vi "Call Matlab Function.vi"(7 "Timestamp":bool, 8 "error in (no error)":errorcluster, 9 "Matlab Param Array":cluster{"Name":string, "Data":variant}[](array[cluster]), 10 "Function name":string="netStartTrial", 11 "TrialBasedExperiment in":refnum<class "MatlabExperiment.lvclass">) -> (0 "error out":errorcluster, 1 "Return value struct":cluster{"Name":string, "Data":variant}[](array[cluster]), 2 "Return value I32":i32, 3 "TrialBasedExperiment out":refnum<class "MatlabExperiment.lvclass">)   [LabVIEW 2010, in "MatlabExperiment.lvclass"]
uses:
  MatlabExperiment.lvclass
  Matlab API/Matlab API.lvlib
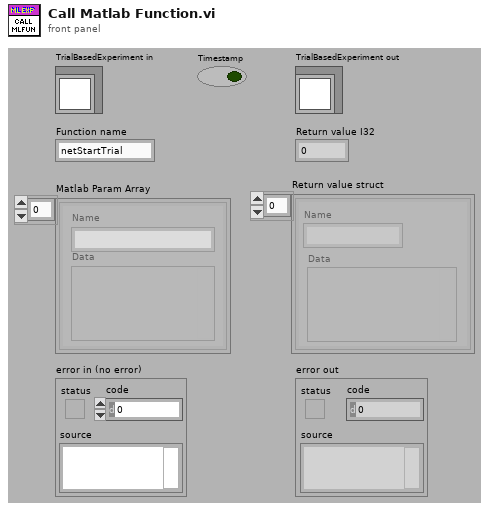
[diagram p1: front panel]
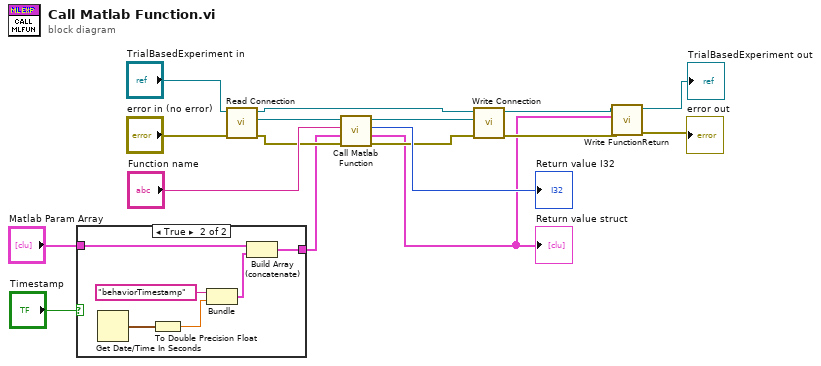
[diagram p0: block diagram]
diagram:
  n1 = case shown="True" "Timestamp" {
    tunnel: "Matlab Param Array" -> [w18 w22]
    tunnel: [w18 w21] -> w7
    frame False {
    }
    frame True {
      n2 = Get Date/Time In Seconds() -> (seconds since 1Jan1904=w20:timestamp)
      n3 = To Double Precision Float(number=w20) -> (double precision float=w19:dbl)
      n4 = Bundle("behaviorTimestamp", w19) -> (w23:cluster{string, dbl})  [unwired: 1 out]
      n5 = Build Array (concatenate)(w22, w23) -> (w21:cluster{"Name":string, "Data":variant}[])
    }
  }
  n6 = call-dynamic "Read Connection.vi"("error in (no error)"="error in (no error)", "TrialBasedExperiment in"="TrialBasedExperiment in") -> ("error out"=w13:errorcluster, "Connection"=w15:refnum<k5>, "TrialBasedExperiment out"=w17:refnum<class "MatlabExperiment.lvclass">)  [unwired: 7 in]
  n7 = call "Call Matlab Function.vi"("error in (no error)"=w13, "Matlab Param Array"=w7, "Function name"="Function name", "TCP Network Connection Refnum"=w15) -> ("error out"=w9:errorcluster, "Return value struct"=w1:cluster{"Name":string, "Data":variant}[], "Return value I32"=→"Return value I32":i32, "connection ID out"=w10:refnum<k5>)  [unwired: 4 out]
  "Return value struct" <- w1
  n8 = call-dynamic "Write Connection.vi"("error in (no error)"=w9, "Connection"=w10, "TrialBasedExperiment in"=w17) -> ("error out"=w4:errorcluster, "TrialBasedExperiment out"=w5:refnum<class "MatlabExperiment.lvclass">)  [unwired: 7 in]
  n9 = call-dynamic "Write FunctionReturn.vi"("error in (no error)"=w4, "FunctionReturn"=w1, "MatlabExperiment in"=w5) -> ("error out"=→"error out":errorcluster, "MatlabExperiment out"=→"TrialBasedExperiment out":refnum<class "MatlabExperiment.lvclass">)  [unwired: 7 in]
